vi "Close.vi"(8 "error in (no error)":errorcluster) -> (0 "error out":errorcluster, 2 "Images":path[](array[path]), 3 "API.md":path)   [LabVIEW 2018, in "Markdown.lvlib"]
doc: "Return the exported markdown and images paths and close the library references."
uses:
  Markdown.lvlib
  Global.vi
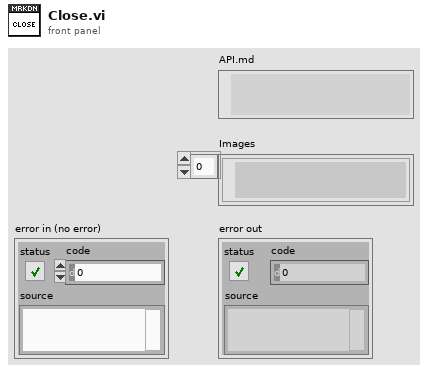
[diagram p1: front panel]
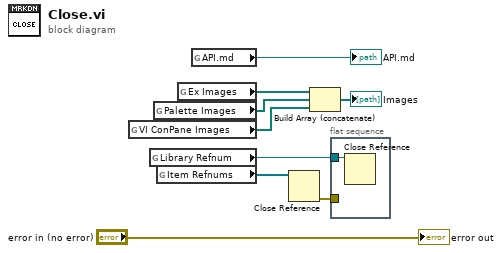
[diagram p0: block diagram]
diagram:
  n1 = global read "Global.vi" "VI ConPane Images"() -> (w3:path[])
  n2 = global read "Global.vi" "Library Refnum"() -> (w2:refnum<vi>)
  n3 = global read "Global.vi" "Palette Images"() -> (w4:path[])
  n4 = global read "Global.vi" "Item Refnums"() -> (w1:refnum<vi>[])
  n5 = global read "Global.vi" "Ex Images"() -> (w5:path[])
  n6 = global read "Global.vi" "API.md"() -> (→"API.md":path)
  n7 = Close Reference(reference=w1) -> (error out=w7:errorcluster)  [unwired: 1 in]
  n8 = Build Array (concatenate)(w5, w4, w3) -> (→"Images":path[])
  n9 = flat-sequence {
    tunnel: w2 -> [w10]
    tunnel: w7 -> [_]
    frame #0 {
      n10 = Close Reference(reference=w10) -> ()  [unwired: 1 in, 1 out]
    }
  }
  "error out" <- "error in (no error)"
